vi "Wait.vi"(8 "error":errorcluster, 10 "Delay (20 mS)":u32=20, 11 "VISA":refnum<visa-resource-name>) -> (0 "error out":errorcluster, 3 "VISA out":refnum<visa-resource-name>)   [LabVIEW 2023, in "TDK-Lambda GEN LAN Series.lvlib"]
doc: "Waits number of milliseconds. Used for allowing instrument to settle after changing the output. If \"Delay\" input not wired, it will wait 20 mSec.\n\nIf \"error\" input is set to error, the VI will not wait."
uses:
  TDK-Lambda GEN LAN Series.lvlib
panel:
  # "TDK-Lambda Genesys \n LAN\n  DC Power Supplies"
  # "WAIT\nmilliSeconds"
  # "(c) 2019 TDK-Lambda.  ALL RIGHTS RESERVED."
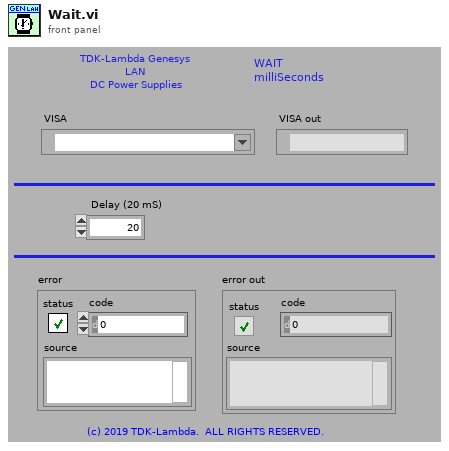
[diagram p1: front panel]
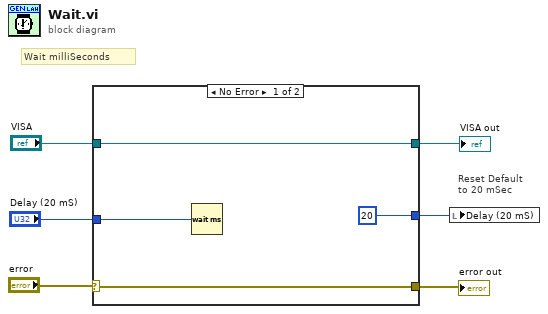
[diagram p0: block diagram]
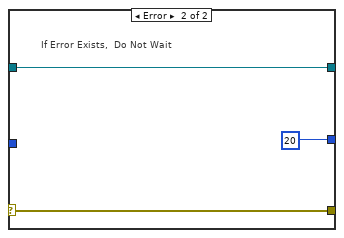
[diagram p2: hidden frame]
diagram:
  # "Reset Default\nto 20 mSec"
  # "Wait milliSeconds"
  n1 = case shown="No Error" "error" {
    selector: "error" -> [w10 w12]
    tunnel: [w10 w12] -> w5
    tunnel: "VISA" -> [w9 w13]
    tunnel: [w9 w13] -> w3
    tunnel: [u32 20 ("Delay (20 mS)") u32 20 ("Delay (20 mS)")] -> w2
    tunnel: "Delay (20 mS)" -> [w7 _]
    frame No Error {
      n2 = Wait (ms)(milliseconds to wait=w7) -> ()  [unwired: 1 out]
    }
    frame Error {
      # "If Error Exists,  Do Not Wait"
    }
  }
  "error out" <- w5
  "VISA out" <- w3
  n3 = local write "Delay (20 mS)"(w2) -> ()
